vi "File to Array.vi"(8 "error in":errorcluster, 11 "file path in":path) -> (0 "error out":errorcluster, 2 "list out":T1[](array[typedef]) {"Last Updated" format="%<%x>T"}, 3 "file path out":path)   [LabVIEW 2018]
uses:
  SR Cluster.ctl
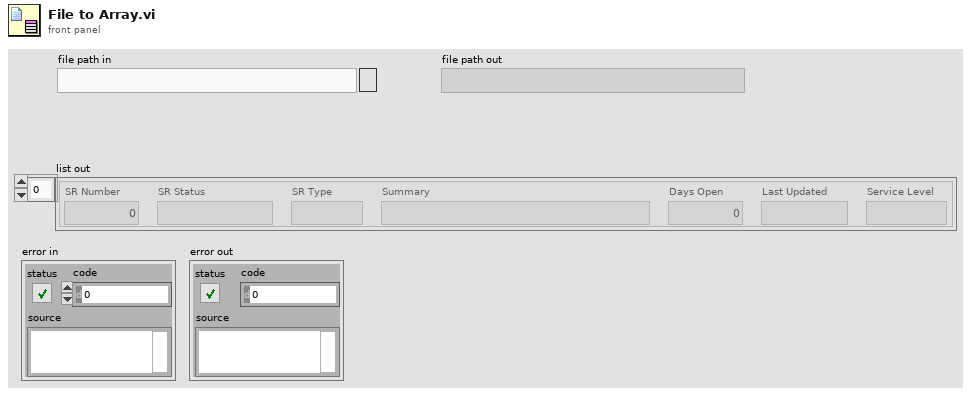
[diagram p1: front panel]
types:
  T1 = typedef "SR Cluster.ctl" = cluster{"SR Number":i32, "SR Status":string, "SR Type":string, "Summary":string, "Days Open":dbl, "Last Updated":timestamp, "Service Level":string}
  T2 = enum16{"open", "replace", "create", "open or create", "replace or create", "replace or create with confirmation"}
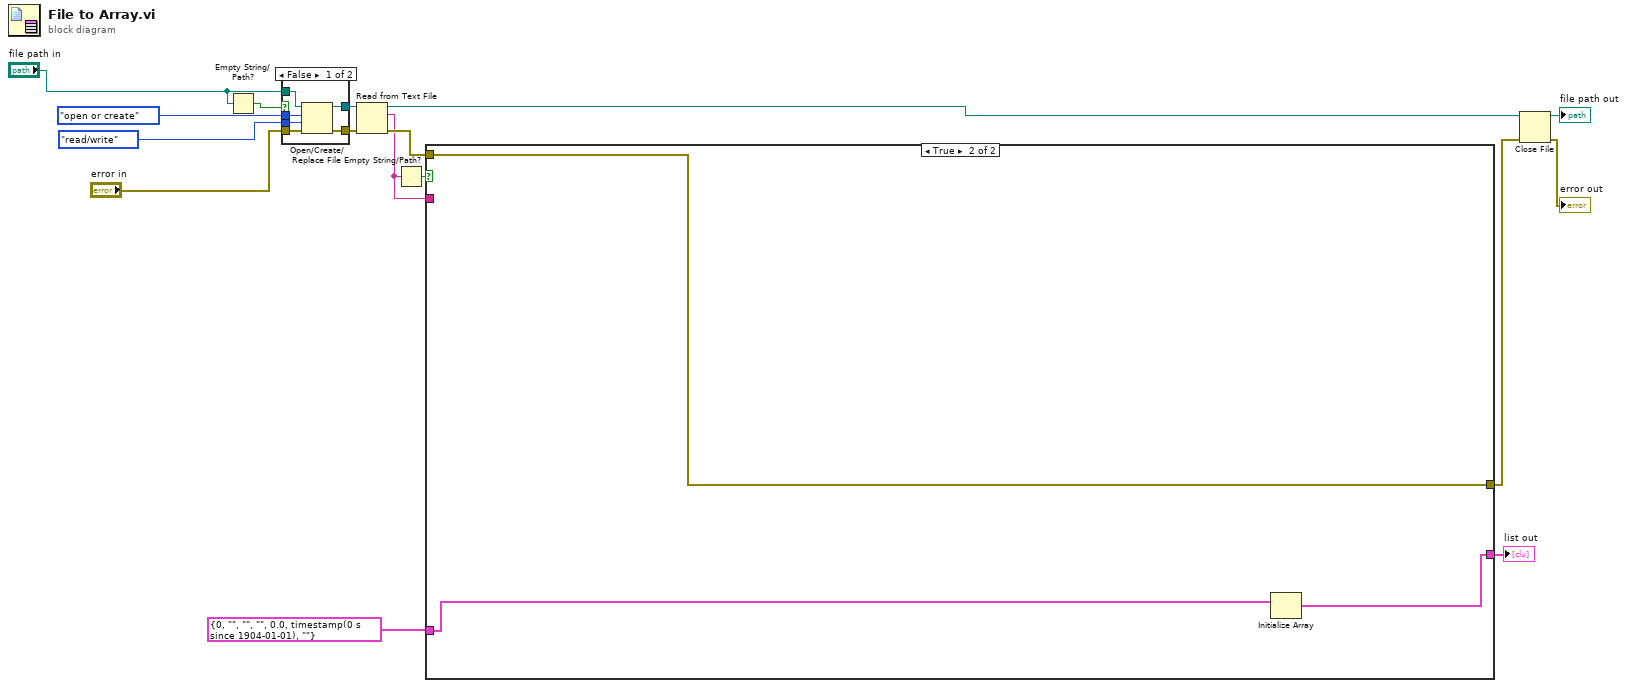
[diagram p0: block diagram]
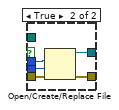
[diagram p2: hidden frame]
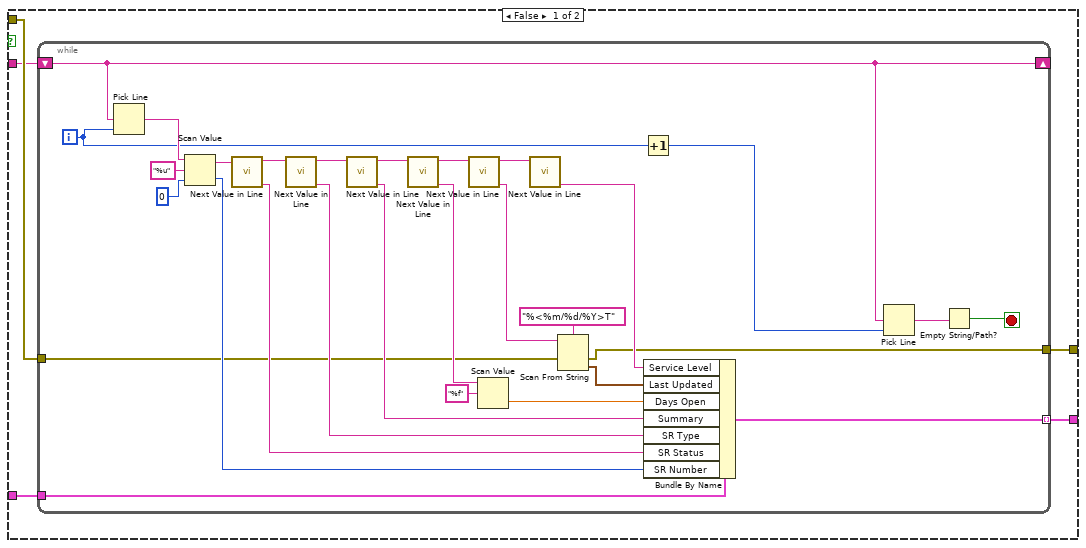
[diagram p3: hidden frame]
diagram:
  n1 = Empty String/Path?(string/path="file path in") -> (empty?=w2:bool)
  n2 = case shown="False" w2 {
    tunnel: enum16{"read/write", "read-only", "write-only"}."read/write" ("access (0:read/write)") -> [w22 w26]
    tunnel: T2."open or create" ("operation (0:open)") -> [w21 w27]
    tunnel: "error in" -> [w20 w25]
    tunnel: [w19 w23] -> w13
    tunnel: [w18 w24] -> w12
    tunnel: "file path in" -> [w17 _]
    frame False {
      n3 = Open/Create/Replace File(file path (use dialog)=w17, error in=w20, operation (0:open)=w21, access (0:read/write)=w22) -> (refnum out=w19:refnum<file>, error out=w18:errorcluster)  [unwired: 2 in, 1 out]
    }
    frame True {
      n4 = Open/Create/Replace File(error in=w25, operation (0:open)=w27, access (0:read/write)=w26) -> (refnum out=w23:refnum<file>, error out=w24:errorcluster)  [unwired: 3 in, 1 out]
    }
  }
  n5 = Read from Text File(file (use dialog)=w13, error in=w12) -> (refnum out=w7:refnum<file>, text=w9:string, error out=w10:errorcluster)  [unwired: 2 in, 1 out]
  n6 = Empty String/Path?(string/path=w9) -> (empty?=w11:bool)
  n7 = case shown="True" w11 {
    tunnel: w10 -> [w31 w62]
    tunnel: w9 -> [w30 _]
    tunnel: T1 {"SR Number"=0, "SR Status"="", "SR Type"="", "Summary"="", "Days Open"=0.0, "Last Updated"=timestamp(0 s since 1904-01-01), "Service Level"=""} ("SR Cluster") -> [w32 w64]
    tunnel: [w29 w62] -> w6
    tunnel: [w28 w63] -> w5
    frame False {
      n8 = while {
        tunnel: w32 -> [w52]
        tunnel: w31 -> [w39]
        shift-right: [w37] -> _
        shift-left: w30 -> [w37]
        tunnel: [w40] -> w28 mode=indexing
        tunnel: [w38] -> w29
        i -> [w34]
        stop <- w35 stop-if-true
        n9 = Pick Line(multi-line string=w37, line index=w34) -> (output string=w61:string)  [unwired: 1 in]
        n10 = Scan Value(string=w61, format string="%u", default (0 dbl)=0) -> (output string=w58:string, value=w51:i32)
        n11 = call "Next Value in Line.vi"("string in"=w58) -> ("value"=w50:string, "rest of string"=w57:string)  [unwired: 9 in]
        n12 = call "Next Value in Line.vi"("string in"=w57) -> ("value"=w49:string, "rest of string"=w56:string)  [unwired: 9 in]
        n13 = call "Next Value in Line.vi"("string in"=w56) -> ("value"=w48:string, "rest of string"=w55:string)  [unwired: 9 in]
        n14 = call "Next Value in Line.vi"("string in"=w55) -> ("value"=w46:string, "rest of string"=w54:string)  [unwired: 9 in]
        n15 = call "Next Value in Line.vi"("string in"=w54) -> ("value"=w44:string, "rest of string"=w53:string)  [unwired: 9 in]
        n16 = Scan Value(string=w46, format string="%f") -> (value=w47:dbl)  [unwired: 1 in, 1 out]
        n17 = call "Next Value in Line.vi"("string in"=w53) -> ("value"=w41:string)  [unwired: 9 in, 1 out]
        n18 = Scan From String(format string="%<%m/%d/%Y>T", input string=w44, error in=w39) -> (error out=w38:errorcluster, output 1=w42:timestamp)  [unwired: 2 in, 2 out]
        n19 = Increment(x=w34) -> (x+1=w33:i32)
        n20 = Bundle By Name(cluster=w52, "Service Level"=w41, "Last Updated"=w42, "Days Open"=w47, "Summary"=w48, "SR Type"=w49, "SR Status"=w50, "SR Number"=w51) -> (w40:T1)
        n21 = Pick Line(multi-line string=w37, line index=w33) -> (output string=w36:string)  [unwired: 1 in]
        n22 = Empty String/Path?(string/path=w36) -> (empty?=w35:bool)
      }
    }
    frame True {
      n23 = Initialize Array(w64) -> (w63:T1[])  [unwired: 1 in]
    }
  }
  "list out" <- w5
  n24 = Close File(refnum=w7, error in=w6) -> (path=→"file path out":path, error out=→"error out":errorcluster)
